vi "Joystick.vi"() -> (2 "Joystick":T1)   [LabVIEW 2016]
uses:
  Global_Var_Drive.vi
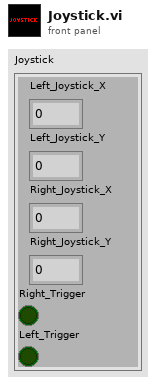
[diagram p1: front panel]
types:
  T1 = cluster{"Left_Joystick_X":dbl, "Left_Joystick_Y":dbl, "Right_Joystick_X":dbl, "Right_Joystick_Y":dbl, "Right_Trigger":bool, "Left_Trigger":bool}
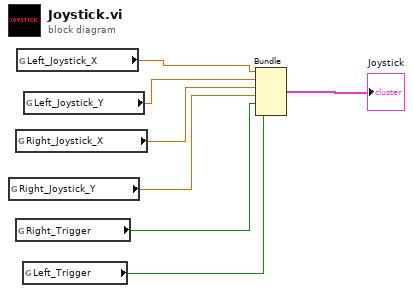
[diagram p0: block diagram]
diagram:
  n1 = global read "Global_Var_Drive.vi" "Right_Joystick_Y"() -> (w4:dbl)
  n2 = global read "Global_Var_Drive.vi" "Right_Joystick_X"() -> (w5:dbl)
  n3 = global read "Global_Var_Drive.vi" "Right_Trigger"() -> (w3:bool)
  n4 = global read "Global_Var_Drive.vi" "Left_Joystick_X"() -> (w7:dbl)
  n5 = global read "Global_Var_Drive.vi" "Left_Trigger"() -> (w2:bool)
  n6 = global read "Global_Var_Drive.vi" "Left_Joystick_Y"() -> (w6:dbl)
  n7 = Bundle("Left_Joystick_X"=w7, "Left_Joystick_Y"=w6, "Right_Joystick_X"=w5, "Right_Joystick_Y"=w4, "Right_Trigger"=w3, "Left_Trigger"=w2) -> (→"Joystick":T1)  [unwired: 1 in]
